vi "Read Job Report Event.vi"(8 "error in (no error)":errorcluster, 11 "Job in":refnum<class "Job.lvclass">) -> (0 "error out":errorcluster, 2 "Job Report Event":refnum<user-event>, 3 "Job out":refnum<class "Job.lvclass">)   [LabVIEW 2013, in "openCronJob.lvlib" / "Job.lvclass"]
uses:
  Job.lvclass
  JobReport/JobReport.lvclass
  Job.lvclass/Job.ctl
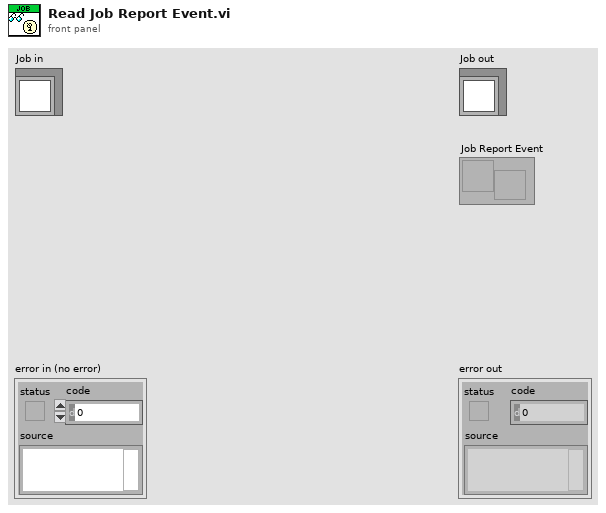
[diagram p1: front panel]
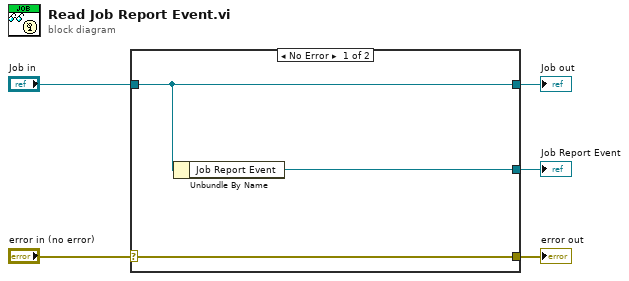
[diagram p0: block diagram]
diagram:
  n1 = case shown="No Error" "error in (no error)" {
    selector: "error in (no error)" -> [w8 w9]
    tunnel: [w8 w9] -> w4
    tunnel: [w7 w10] -> w2
    tunnel: "Job in" -> [w7 w10]
    tunnel: [w6 _] -> w1
    frame No Error {
      n2 = Unbundle By Name(w7) -> ("Job Report Event"=w6:refnum<user-event>)
    }
    frame Error {
    }
  }
  "error out" <- w4
  "Job out" <- w2
  "Job Report Event" <- w1
